vi "State Right value from Ref.vi"(8 "error in (no error)":errorcluster, 10 "States":T1, 11 "Display Panel.lvlib:Abstract Display.lvclass":refnum<class "Abstract Display.lvclass">) -> (0 "error out":errorcluster, 3 "Abstract Display out":refnum<class "Abstract Display.lvclass">)   [LabVIEW 2014, in "Display Panel.lvlib" / "Abstract Display.lvclass"]
uses:
  Abstract Display.lvclass
  State.ctl
  Abstract Display.lvclass/Abstract Display.ctl
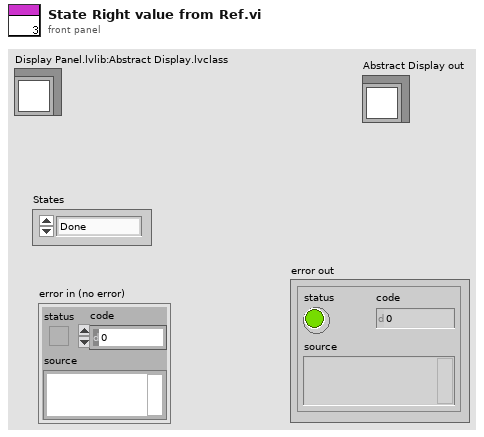
[diagram p1: front panel]
types:
  T1 = typedef "Display Panel.lvlib/Abstract Display.lvclass/State.ctl" = enum16{"Done", "Warming", "Measuring"}
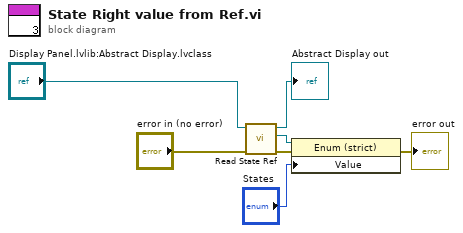
[diagram p0: block diagram]
diagram:
  n1 = call "Read State Ref.vi"("error in (no error)"="error in (no error)", "Abstract Display in"="Display Panel.lvlib:Abstract Display.lvclass") -> ("error out"=w5:errorcluster, "State Ref"=w6:refnum<vi>, "Abstract Display out"=→"Abstract Display out":refnum<class "Abstract Display.lvclass">)  [unwired: 7 in]
  n2 = property class="Enum (strict)"(reference=w6, error in=w5, "Value"="States") -> (error out=→"error out":errorcluster)  [unwired: 1 out]
